vi "CTRE_Phoenix_CANifier_SetStatusFramePeriod.vi"(6 "timeoutMs":i32, 8 "error in (no error)":errorcluster, 9 "periodMs":i32, 10 "CANifier Status Frame":T1=267264 items=["Status_1_General"=267264, "Status_2_General"=267328, "Status_3_PwmInputs0"=267392, "Status_4_PwmInputs1"=267456, "Status_5_PwmInputs2"=267520, "Status_6_PwmInputs3"=267584, "Status_8_Misc"=267712], 11 "CANifierDevRef":T2) -> (0 "error out":errorcluster, 3 "CANifierDevRef":T2)   [LabVIEW 2017]
doc: "Set the period of the specified status frame."
uses:
  CTRE_CANifier_DeviceRef.ctl
  CTRE_CANifier_StatusFrame.ctl
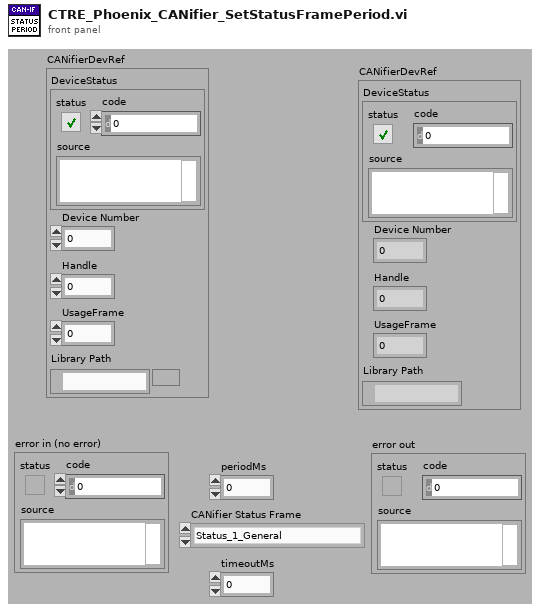
[diagram p1: front panel]
types:
  T1 = typedef "CTRE_CANifier_StatusFrame.ctl" = u32
  T2 = typedef "CTRE_CANifier_DeviceRef.ctl" = cluster{"DeviceStatus":errorcluster, "Device Number":u8, "Handle":u64, "UsageFrame":u32, "Library Path":path}
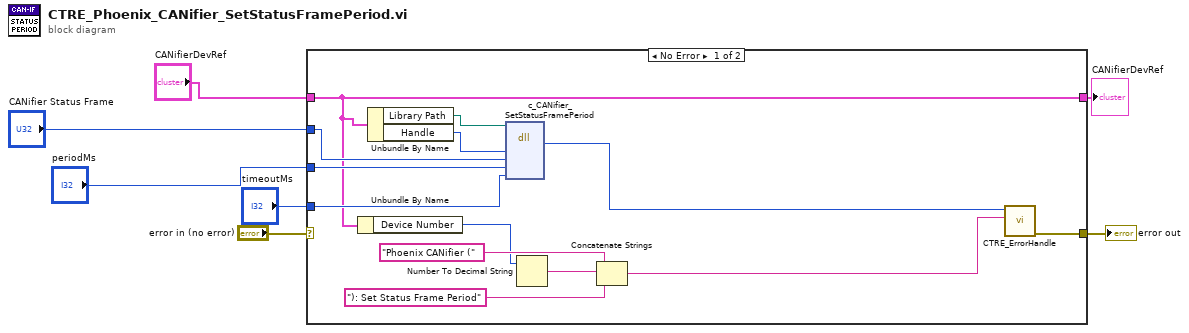
[diagram p0: block diagram]
diagram:
  n1 = case shown="No Error" "error in (no error)" {
    selector: "error in (no error)" -> [_ w22]
    tunnel: [w17 w22] -> w7
    tunnel: "CANifierDevRef" -> [w10 w21]
    tunnel: [w10 w21] -> w2
    tunnel: "periodMs" -> [w14 _]
    tunnel: "timeoutMs" -> [w13 _]
    tunnel: "CANifier Status Frame" -> [w12 _]
    frame No Error {
      n2 = Unbundle By Name(w10) -> ("Device Number"=w11:u8)
      n3 = Unbundle By Name(w10) -> ("Library Path"=w9:path, "Handle"=w8:u64)
      n4 = dll-call lib="?" fn="c_CANifier_SetStatusFramePeriod"(path in=w9, "handle"=w8, "frame"=w12, "periodMs"=w14, "timeoutMs"=w13) -> ("ErrorCode"=w15:i32)  [unwired: 6 in, 2 out]
      n5 = Number To Decimal String(number=w11) -> (decimal integer string=w19:string)  [unwired: 1 in]
      n6 = Concatenate Strings("Phoenix CANifier (" ("string"), w19, "): Set Status Frame Period" ("string")) -> (w16:string)
      n7 = call "CTRE_ErrorHandle.vi"("origin"=w16, "code"=w15) -> ("error out"=w17:errorcluster)  [unwired: 9 in]
    }
    frame Error {
    }
  }
  "error out" <- w7
  "CANifierDevRef" <- w2
